vi "turnLaserOn.vi"(1 "input cluster":T1) -> (0 "laser on":bool)   [LabVIEW 2015]
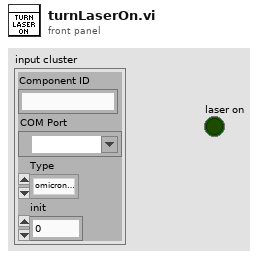
[diagram p1: front panel]
types:
  T1 = cluster{"Component ID":string, "COM Port":refnum<visa-resource-name>, "Type ":enum16{"omicronLuxX", "coherentObis"}, "init":i16}
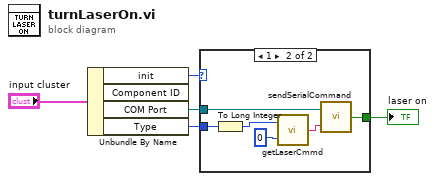
[diagram p0: block diagram]
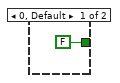
[diagram p2: hidden frame]
diagram:
  n1 = Unbundle By Name("input cluster") -> ("init"=w3:i16, "COM Port"=w4:refnum<visa-resource-name>, "Type"=w5:enum16{"omicronLuxX", "coherentObis"})  [unwired: 1 out]
  n2 = case shown="1" w3 {
    tunnel: w4 -> [_ w11]
    tunnel: w5 -> [_ w8]
    tunnel: [FALSE ("data written to port?") w9] -> w1
    frame 0, Default {
    }
    frame 1 {
      n3 = To Long Integer(number=w8) -> (32bit integer=w7:i32)
      n4 = call "getLaserCmmd.vi"("Cmmd index"=0, "Laser type"=w7) -> ("Laser command"=w10:string)
      n5 = call "sendSerialCommand.vi"("Cmmd"=w10, "input COM Port"=w11) -> ("data written to port?"=w9:bool)
    }
  }
  "laser on" <- w1
